vi "IsProcessRunning.vi"(8 "error in (no error)":errorcluster, 10 "Kill if running? (F)":bool, 11 "Program Name":string) -> (0 "error out":errorcluster, 3 "Running?":bool)   [LabVIEW 2019, in "Tools.lvlib"]
doc: "Check if an exe is running and optionally kill the process"
uses:
  Tools.lvlib
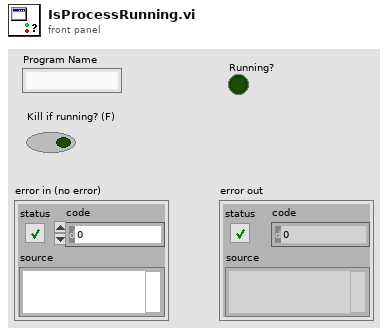
[diagram p1: front panel]
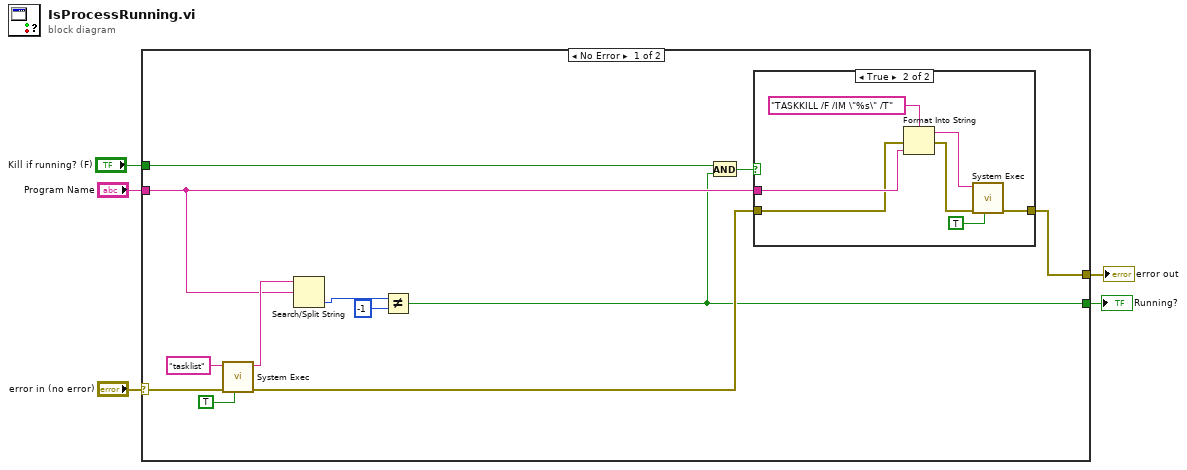
[diagram p0: block diagram]
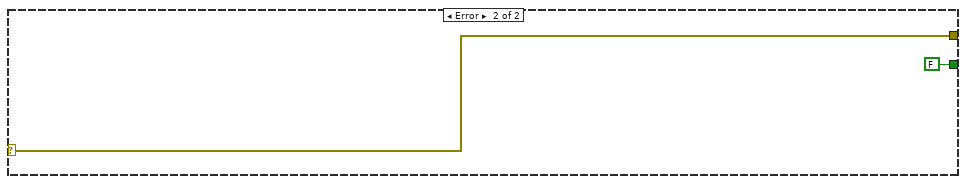
[diagram p3: hidden frame]
diagram:
  n1 = case shown="No Error" "error in (no error)" {
    selector: "error in (no error)" -> [w12 w27]
    tunnel: [w6 FALSE] -> w5
    tunnel: "Program Name" -> [w9 _]
    tunnel: [w15 w27] -> w3
    tunnel: "Kill if running? (F)" -> [w17 _]
    frame No Error {
      n2 = call <vilib>:"System Exec.vi"("run minimized? (F)"=TRUE, "error in (no error)"=w12, "command line"="tasklist" ("standard input")) -> ("error out"=w11:errorcluster, "standard output"=w10:string)  [unwired: 5 in, 2 out]
      n3 = Search/Split String(string=w10, search string/char (-)=w9) -> (offset of match=w8:i32)  [unwired: 1 in, 2 out]
      n4 = Not Equal?(x=w8, y=-1) -> (x != y?=w6:bool)
      n5 = And(x=w17, y=w6) -> (x .and. y?=w16:bool)
      n6 = case shown="True" w16 {
        tunnel: w9 -> [_ w24]
        tunnel: w11 -> [w18 w20]
        tunnel: [w18 w25] -> w15
        frame False {
        }
        frame True {
          n7 = Format Into String(format string="TASKKILL /F /IM \"%s\" /T", error in=w20, w24) -> (resulting string=w22:string, error out=w21:errorcluster)  [unwired: 1 in]
          n8 = call <vilib>:"System Exec.vi"("run minimized? (F)"=TRUE, "error in (no error)"=w21, "command line"=w22) -> ("error out"=w25:errorcluster)  [unwired: 5 in, 3 out]
        }
      }
    }
    frame Error {
    }
  }
  "Running?" <- w5
  "error out" <- w3
